vi "Protocol.Process Incoming Messages by PDU F.vi"(6 "State":T1=enum."ACL", 8 "error in":errorcluster, 10 "CAN frame":T2 {"payload" format="%x"; "timestamp" format="%<%.7X\n%x>T"; "type" items=["CAN Data"=0, "CAN Remote"=1, "CAN Bus Error"=2, "CAN 2.0 Data"=8, "CAN FD Data"=16, "CAN FD+BRS Data"=24, "J1939 Data"=192, "Delay"=224, "Log Trigger"=225, "Start Trigger"=226]; "identifier" format="%x"}, 11 "J1939 Cluster":T4) -> (0 "error out":errorcluster)   [LabVIEW 2023, in "J1939 Addon Engine.lvlib"]
uses:
  J1939 Addon Engine.lvlib
  Types/Protocol.Refs.ctl
  Support Libraries/J1939 Utilities/Types/CAN Outgoing Message Cluster.ctl
  Types/Protocol.RQST Lookup Table Reference.ctl
  Types/Protocol.Address Table Reference.ctl
  <vilib>/xnet/xnet.llb/XNET Frame CAN.ctl
  <vilib>/xnet/xnet.llb/XNET Frame Type CAN.ctl
  Support Libraries/J1939 Utilities/Types/Message Types.ctl
  Types/Protocol.RQST Lookup Table Action.ctl
  Types/Engine.Node DTC Settings.ctl
  Addon Shared/Types/Monitor Settings.ctl
  Types/Engine.DTC Settings.ctl
  Addon Shared/Types/Compiled Simulated Settings.ctl
  <vilib>/NI VeriStand/Custom Device API/Block Data Reference.ctl
  <vilib>/NI VeriStand/Custom Device API/Data Reference.ctl
  Types/Engine.DTC FIFOs.ctl
  Support Libraries/J1939 Utilities/Types/PGN Fields Cluster.ctl
  Types/Protocol.Address Lookup Table Action.ctl
  Addon Shared/Types/Address Lookup Table Data.ctl
  Support Libraries/J1939 Utilities/SubVIs/Convert CAN Arb ID to J1939 ID.vi
  Support Libraries/J1939 Utilities/SubVIs/Convert J1939 ID to CAN Arb ID.vi
  Support Libraries/J1939 Utilities/SubVIs/Convert CAN Data (U32) to U8.vi
  Support Libraries/J1939 Utilities/SubVIs/Acknowledgement.vi
  Protocol.Convert Data to DTC Frame.vi
  Protocol.RQST Lookup Table.vi
  <vilib>/xnet/xnet.llb/XNET Create Session.vi
  <vilib>/xnet/xnet.llb/XNET Create Session (Conversion).vi
  <vilib>/xnet/xnet.llb/XNET Convert.vi
  <vilib>/xnet/xnet.llb/XNET Convert (Signal to Frame CAN).vi
  <vilib>/xnet/xnet.llb/XNET Clear.vi
  Protocol.Address Lookup Table.vi
  Support Libraries/J1939 Utilities/J1939 Utilities.lvlib
  <vilib>/NI VeriStand/Custom Device API/Custom Device API.lvlib
  Addon Shared/J1939 Addon Shared.lvlib
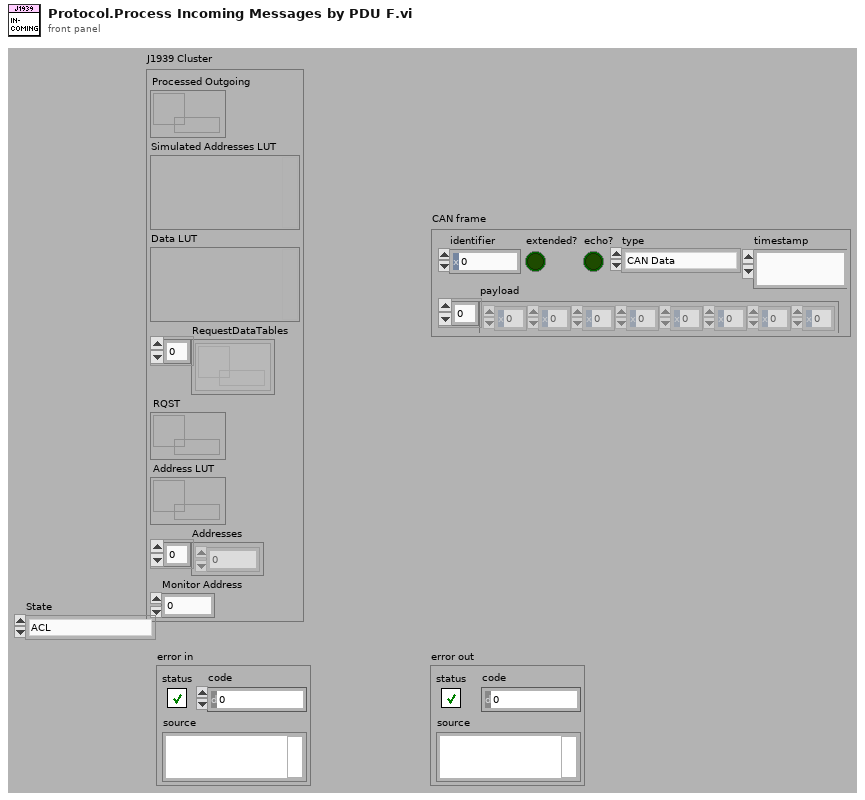
[diagram p1: front panel]
types:
  T1 = typedef "J1939 Utilities.lvlib/Message Types.ctl" = enum8{"PDU 1", "RQST2", "XFER", "ACKM", "RQST", "TP.DT - RTS/CTS", "TP.DT - BAM", "TP.CM - RTS", "TP.CM - CTS", "TP.CM - EndofMsgACK", "TP.CM - BAM", "TP.CM - Abort", "TP.CM - Error", "ACL", "Proprietary A", "PDU 2", "Proprietary B", "Error"}
  T2 = typedef "XNET Frame CAN.ctl" = cluster{"timestamp":timestamp, "payload":u8[], "identifier":u32, "type":T3, "extended?":bool, "echo?":bool}
  T3 = typedef "XNET Frame Type CAN.ctl" = u8
  T4 = typedef "J1939 Addon Engine.lvlib/Protocol.Refs.ctl" = cluster{"Processed Outgoing":refnum<queue>, "Simulated Addresses LUT":variant, "Data LUT":variant, "RequestDataTables":refnum<k33>[], "RQST":T5, "Address LUT":T6, "Addresses":u8[], "Monitor Address":u8}
  T5 = typedef "J1939 Addon Engine.lvlib/Protocol.RQST Lookup Table Reference.ctl" = refnum<data-value>
  T6 = typedef "J1939 Addon Engine.lvlib/Protocol.Address Table Reference.ctl" = refnum<data-value>
  T7 = typedef "J1939 Addon Engine.lvlib/Protocol.RQST Lookup Table Action.ctl" = enum16{"Initialize", "Add", "Get", "Remove", "Get Active Requests"}
  T8 = typedef "J1939 Addon Engine.lvlib/Engine.Node DTC Settings.ctl" = cluster{"Network":T9, "Sim DTC Refs":T10}
  T9 = typedef "J1939 Addon Shared.lvlib/Monitor Settings.ctl" = cluster{"Address":u8, "Name":u64, "Include DA":bool, "Force SA":bool}
  T10 = typedef "J1939 Addon Engine.lvlib/Engine.DTC Settings.ctl" = cluster{"Data":T11, "FIFOs":T14}
  T11 = typedef "J1939 Addon Shared.lvlib/Compiled Simulated Settings.ctl" = cluster{"DM1.Ref":T12[], "DM1.Value":dbl[], "DM1.Enable.Ref":T12[], "DM1.Enable.Value":dbl[], "DM2.Ref":T12[], "DM2.Value":dbl[], "DM2.Enable.Ref":T12[], "DM2.Enable.Value":dbl[]}
  T12 = typedef "Custom Device API.lvlib/Block Data Reference.ctl" = cluster{"Data Reference":T13, "Offset":u64, "Length":u64}
  T13 = typedef "Custom Device API.lvlib/Data Reference.ctl" = i32
  T14 = typedef "J1939 Addon Engine.lvlib/Engine.DTC FIFOs.ctl" = cluster{"DM1.Data":refnum<k33>, "DM1.Enable":refnum<k33>, "DM2.Data":refnum<k33>, "DM2.Enable":refnum<k33>, "DM1.Reset":refnum<k33>, "DM2.Reset":refnum<k33>}
  T15 = typedef "J1939 Utilities.lvlib/PGN Fields Cluster.ctl" = cluster{"Reserved Bit":u8, "Data page":u8, "PDU Format":u8, "PDU Specific":u8}
  T16 = typedef "J1939 Utilities.lvlib/CAN Outgoing Message Cluster.ctl" = cluster{"Identifier":u32, "Data":u8[]}
  T17 = typedef "J1939 Addon Engine.lvlib/Protocol.Address Lookup Table Action.ctl" = enum16{"Initialize", "Add", "Get", "Remove", "Get All"}
  T18 = typedef "J1939 Addon Shared.lvlib/Address Lookup Table Data.ctl" = cluster{"Name":u8[], "Address":u8}
  T19 = typedef "J1939 Addon Engine.lvlib/Protocol.RQST Lookup Table Cluster.ctl" = cluster{"Response Q":refnum<queue>, "Request PGN":u32}
  T20 = typedef "J1939 Utilities.lvlib/Convert CAN Data (U8) Cluster.ctl" = cluster{"Byte 1":u8, "Byte 2":u8, "Byte 3":u8, "Byte 4":u8, "Byte 5":u8, "Byte 6":u8, "Byte 7":u8, "Byte 8":u8}
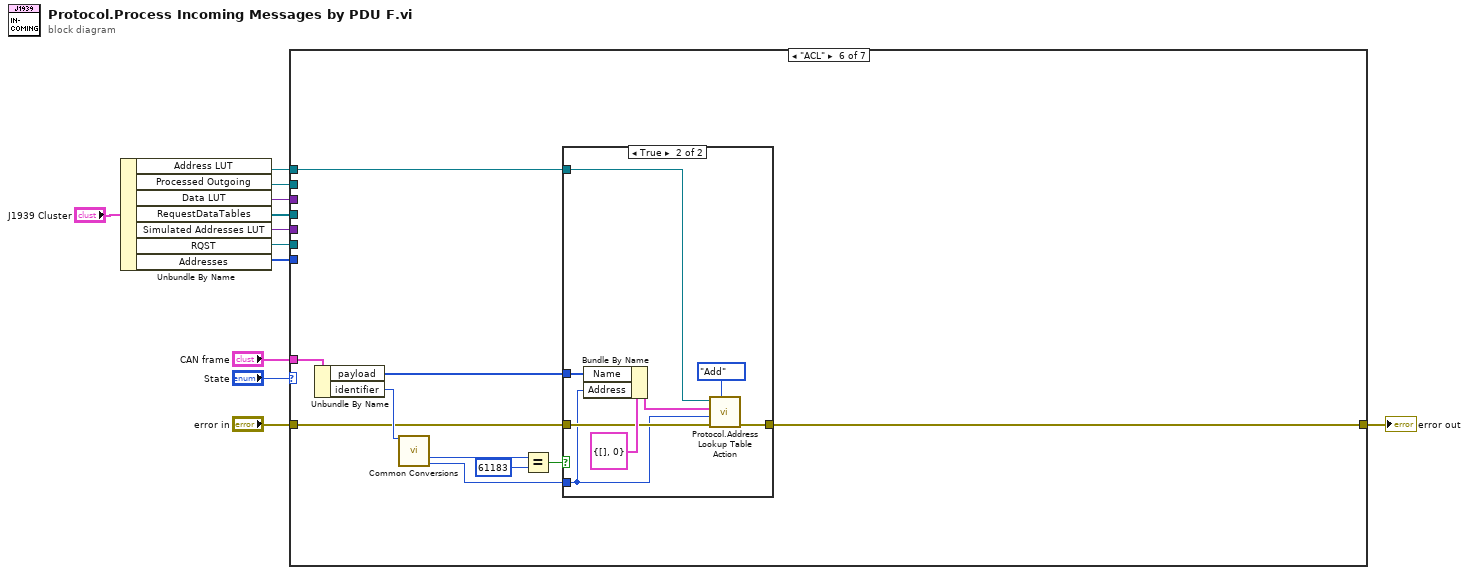
[diagram p0: block diagram]
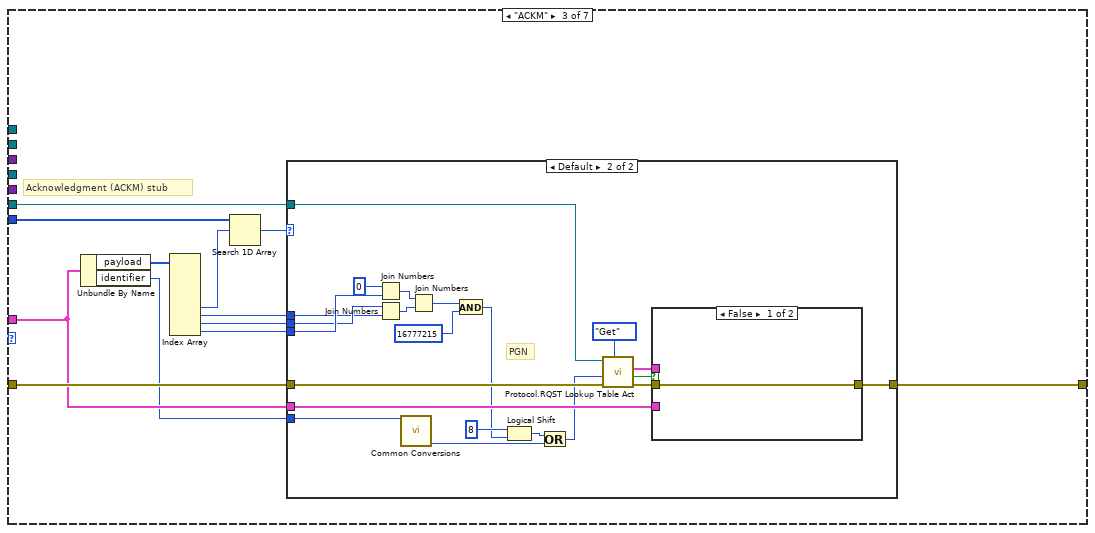
[diagram p4: hidden frame]
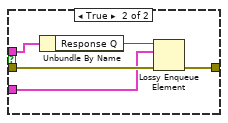
[diagram p6: hidden frame]
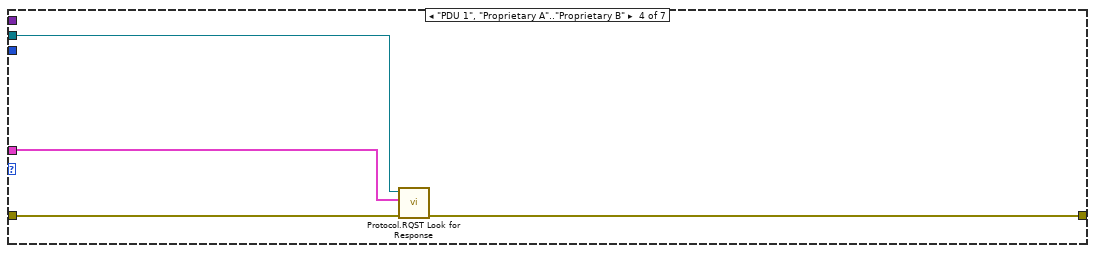
[diagram p7: hidden frame]
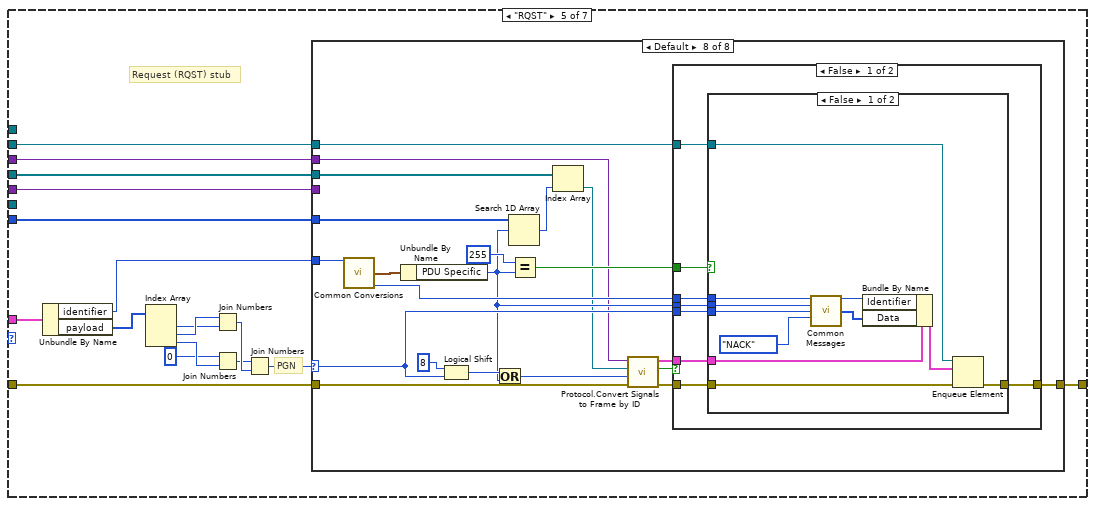
[diagram p8: hidden frame]
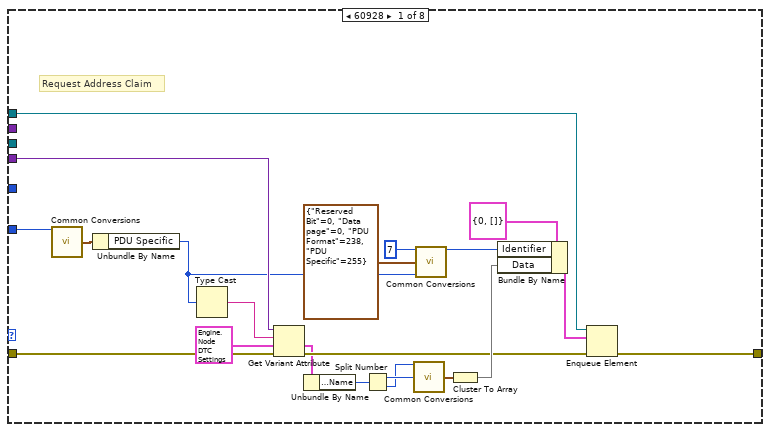
[diagram p9: hidden frame]
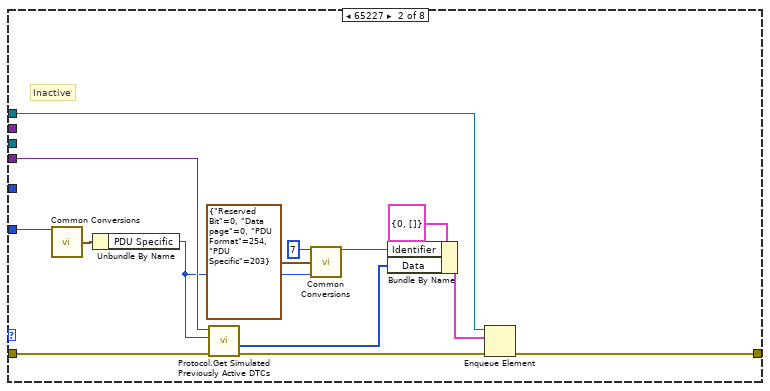
[diagram p10: hidden frame]
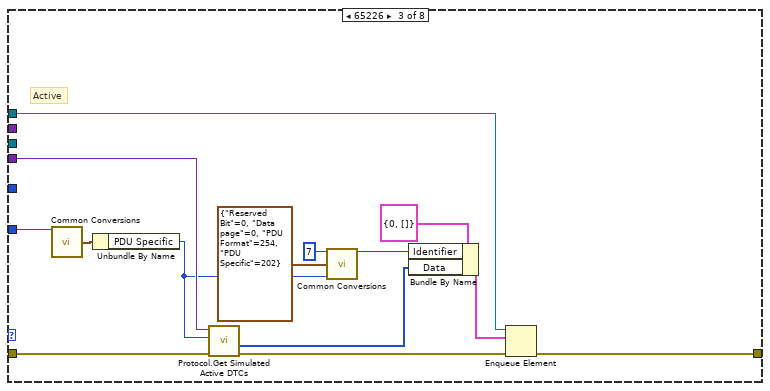
[diagram p11: hidden frame]
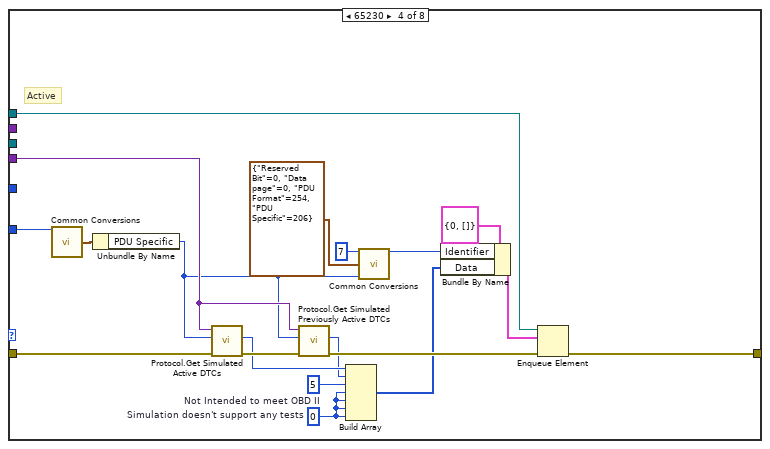
[diagram p12: hidden frame]
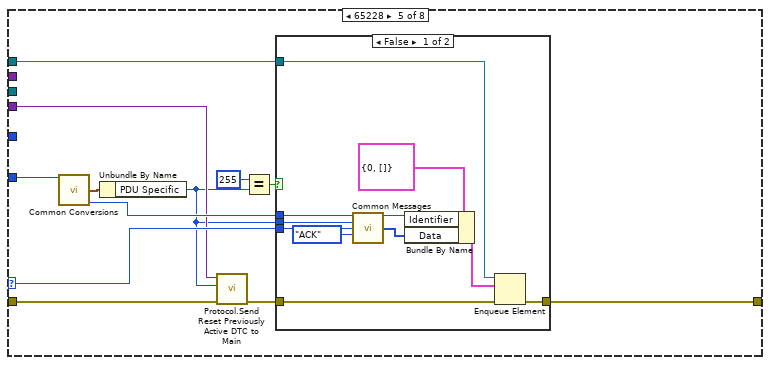
[diagram p13: hidden frame]
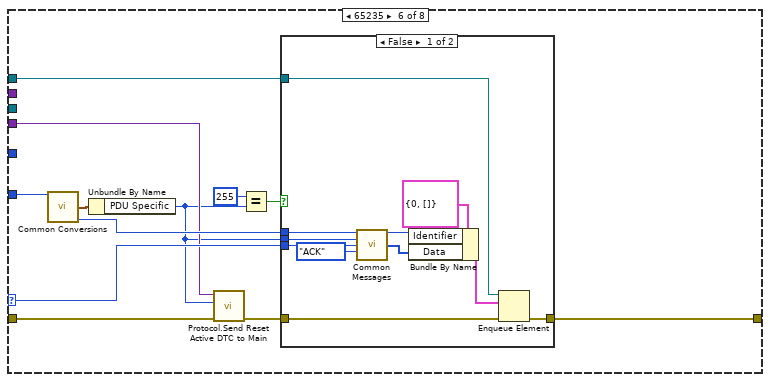
[diagram p15: hidden frame]
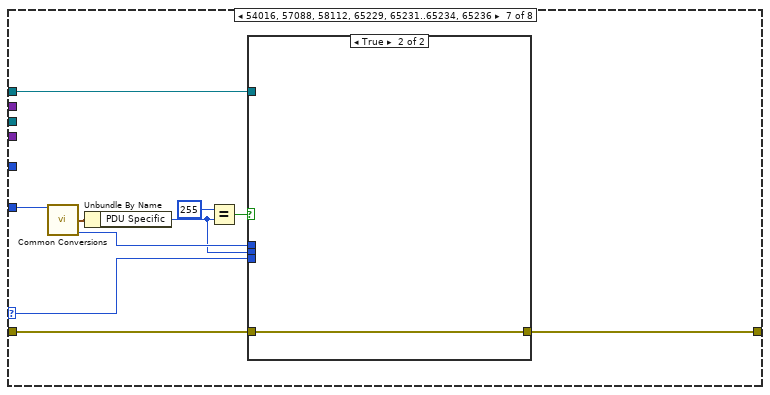
[diagram p17: hidden frame]
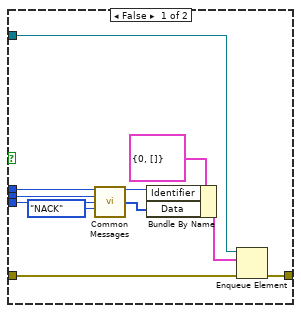
[diagram p18: hidden frame]
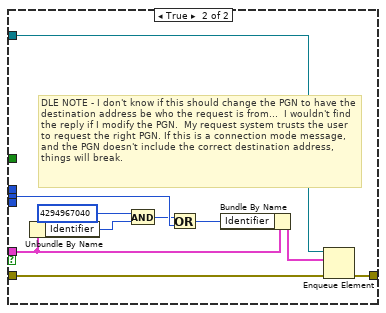
[diagram p20: hidden frame]
diagram:
  n1 = Unbundle By Name("J1939 Cluster") -> ("Address LUT"=w1:T6, "Processed Outgoing"=w6:refnum<queue>, "Data LUT"=w9:variant, "RequestDataTables"=w8:refnum<k33>[], "Simulated Addresses LUT"=w7:variant, "RQST"=w10:T5, "Addresses"=w5:u8[])
  n2 = case shown="\"ACL\"" "State" {
    tunnel: "error in" -> [w13 w14 w21 w59 w67 w269 w285]
    tunnel: [w13 w14 w22 w57 w68 w268 w285] -> w12
    tunnel: "CAN frame" -> [_ _ w20 w58 w76 w270 _]
    tunnel: w6 -> [_ _ _ _ w66 _ _]
    tunnel: w10 -> [_ _ w18 w56 _ _ _]
    tunnel: w5 -> [_ _ w17 _ w61 _ _]
    tunnel: w7 -> [_ _ _ _ w63 _ _]
    tunnel: w8 -> [_ _ _ _ w62 _ _]
    tunnel: w9 -> [_ _ _ _ w60 _ _]
    tunnel: w1 -> [_ _ _ _ _ w266 _]
    frame "RQST2" {
      # "Request2 (RQST2) Stub"
    }
    frame "XFER" {
      # "Transfer (XFER) Stub"
    }
    frame "ACKM" {
      # "Acknowledgment (ACKM) stub"
      n3 = Unbundle By Name(w20) -> ("payload"=w26:u8[], "identifier"=w19:u32)
      n4 = Index Array(array=w26) -> (element #5=w16:u8, element #6=w23:u8, element #7=w24:u8, element #8=w25:u8)  [unwired: 8 in, 4 out]
      n5 = Search 1D Array(1D array=w17, element=w16) -> (index of element=w15:i32)  [unwired: 1 in]
      n6 = case shown="Default" w15 {
        tunnel: w25 -> [_ w49]
        tunnel: w24 -> [_ w48]
        tunnel: w23 -> [_ w47]
        tunnel: [w27 w39] -> w22
        tunnel: w21 -> [w27 w38]
        tunnel: w20 -> [_ w37]
        tunnel: w19 -> [_ w34]
        tunnel: w18 -> [_ w29]
        frame -1 {
        }
        frame Default {
          # "PGN"
          n7 = Join Numbers(hi=u8 0, lo=w49) -> ((hi.lo)=w46:u16)
          n8 = Join Numbers(hi=w48, lo=w47) -> ((hi.lo)=w45:u16)
          n9 = call-poly "Common Conversions.vi"("Arb ID"=w34) -> ("Source Address"=w33:u8)  [unwired: 11 in, 3 out]
          n10 = Join Numbers(hi=w46, lo=w45) -> ((hi.lo)=w44:u32)
          n11 = And(x=w44, y=u32 16777215 ("x")) -> (x .and. y?=w32:u32)
          n12 = Logical Shift(y=i8 8, x=w32) -> (x << y=w36:u32)
          n13 = Or(x=w36, y=w33) -> (x .or. y?=w31:u32)
          n14 = call "Protocol.RQST Lookup Table Act.vi"("Action"=Protocol.RQST_Lookup_Table_Action."Get", "error in (no error)"=w38, "ID"=w31, "Rqst LUT"=w29) -> ("error out"=w30:errorcluster, "Found?"=w41:bool, "Data"=w40:T19)  [unwired: 3 in, 2 out]
          n15 = case shown="False" w41 {
            tunnel: w40 -> [_ w54]
            tunnel: w30 -> [w50 w55]
            tunnel: w37 -> [_ w52]
            tunnel: [w50 w51] -> w39
            frame False {
            }
            frame True {
              n16 = Unbundle By Name(w54) -> ("Response Q"=w53:refnum<queue>)
              n17 = Lossy Enqueue Element(queue=w53, element=w52, error in (no error)=w55) -> (error out=w51:errorcluster)  [unwired: 3 out]
            }
          }
        }
      }
    }
    frame "PDU 1", "Proprietary A".."Proprietary B" {
      n18 = call "Protocol.RQST Look for Response.vi"("error in (no error)"=w59, "CAN frame"=w58, "ref in"=w56) -> ("error out"=w57:errorcluster)  [unwired: 8 in]
    }
    frame "RQST" {
      # "PGN"
      # "Request (RQST) stub"
      n19 = Unbundle By Name(w76) -> ("identifier"=w65:u32, "payload"=w75:u8[])
      n20 = Index Array(array=w75) -> (element #1=w64:u8, element #2=w74:u8, element #3=w73:u8)  [unwired: 3 in]
      n21 = Join Numbers(hi=w74, lo=w64) -> ((hi.lo)=w71:u16)
      n22 = Join Numbers(hi=u8 0, lo=w73) -> ((hi.lo)=w70:u16)
      n23 = Join Numbers(hi=w70, lo=w71) -> ((hi.lo)=w69:u32)
      n24 = case shown="Default" w69 {
        selector: w69 -> [_ _ _ _ w150 w175 w197 w227]
        tunnel: [w93 w104 w119 w138 w151 w173 w195 w228] -> w68
        tunnel: w67 -> [w81 w100 w113 w135 w148 w170 w193 w235]
        tunnel: w66 -> [w91 w103 w118 w137 w152 w176 w198 w229]
        tunnel: w65 -> [w85 w110 w124 w143 w155 w174 w196 w230]
        tunnel: w63 -> [w83 w102 w115 w132 w146 w172 _ _]
        tunnel: w62 -> [_ _ _ _ _ _ _ w218]
        tunnel: w61 -> [_ _ _ _ _ _ _ w220]
        tunnel: w60 -> [_ _ _ _ _ _ _ w215]
        frame 60928 {
          # "Request Address Claim"
          n25 = call-poly "Common Conversions.vi"("Arb ID"=w85) -> ("PGN Fields"=w86:T15)  [unwired: 11 in, 3 out]
          n26 = Unbundle By Name(w86) -> ("PDU Specific"=w82:u8)
          n27 = Type Cast(x=w82) -> (*(type *) &x=w84:string)  [unwired: 1 in]
          n28 = Get Variant Attribute(Variant=w83, name=w84, default value (empty Variant)=T8 {"Network"={"Address"=0, "Name"=0, "Include DA"=FALSE, "Force SA"=FALSE}, "Sim DTC Refs"={"Data"={"DM1.Ref"=[], "DM1.Value"=[], "DM1.Enable.Ref"=[], "DM1.Enable.Value"=[], "DM2.Ref"=[], "DM2.Value"=[], "DM2.Enable.Ref"=[], "DM2.Enable.Value"=[]}, "FIFOs"={"DM1.Data"=refnum, "DM1.Enable"=refnum, "DM2.Data"=refnum, "DM2.Enable"=refnum, "DM1.Reset"=refnum, "DM2.Reset"=refnum}}} ("cluster"), error in=w81) -> (value=w79:T8, error out=w80:errorcluster)  [unwired: 2 out]
          n29 = Unbundle By Name(w79) -> ("Network.Name"=w78:u64)
          n30 = Split Number(x=w78) -> (hi(x)=w89:u32, lo(x)=w88:u32)
          n31 = call-poly "Common Conversions.vi"("Data 0-3"=w88, "Data 4-7"=w89) -> ("Byte Cluster"=w90:T20)  [unwired: 13 in]
          n32 = call-poly "Common Conversions.vi"("Priority"=u8 7, "PGN Fields"=T15 {"Reserved Bit"=0, "Data page"=0, "PDU Format"=238, "PDU Specific"=255}, "Source Address"=w82) -> ("ID"=w95:u32)  [unwired: 2 in, 10 out]
          n33 = Cluster To Array(cluster=w90) -> (array=w87:u8[])
          n34 = Bundle By Name(cluster=T16 {"Identifier"=0, "Data"=[]} ("Data to Send"), "Identifier"=w95, "Data"=w87) -> (w92:T16)
          n35 = Enqueue Element(queue=w91, element=w92, error in (no error)=w80) -> (error out=w93:errorcluster)  [unwired: 1 in, 2 out]
        }
        frame 65227 {
          # "Inactive"
          n36 = call-poly "Common Conversions.vi"("Arb ID"=w110) -> ("PGN Fields"=w111:T15)  [unwired: 11 in, 3 out]
          n37 = Unbundle By Name(w111) -> ("PDU Specific"=w101:u8)
          n38 = call "Protocol.Get Simulated Previously Active DTCs.vi"("error in (no error)"=w100, "Address"=w101, "Simulated Addresses LUT"=w102) -> ("error out"=w99:errorcluster, "DTC Frame"=w98:u8[])  [unwired: 5 in, 2 out]
          n39 = call-poly "Common Conversions.vi"("Priority"=u8 7, "PGN Fields"=T15 {"Reserved Bit"=0, "Data page"=0, "PDU Format"=254, "PDU Specific"=203}, "Source Address"=w101) -> ("ID"=w107:u32)  [unwired: 2 in, 10 out]
          n40 = Bundle By Name(cluster=T16 {"Identifier"=0, "Data"=[]} ("Data to Send"), "Identifier"=w107, "Data"=w98) -> (w109:T16)
          n41 = Enqueue Element(queue=w103, element=w109, error in (no error)=w99) -> (error out=w104:errorcluster)  [unwired: 1 in, 2 out]
        }
        frame 65226 {
          # "Active"
          n42 = call-poly "Common Conversions.vi"("Arb ID"=w124) -> ("PGN Fields"=w125:T15)  [unwired: 11 in, 3 out]
          n43 = Unbundle By Name(w125) -> ("PDU Specific"=w114:u8)
          n44 = call "Protocol.Get Simulated Active DTCs.vi"("error in (no error)"=w113, "Address"=w114, "Simulated Addresses LUT"=w115) -> ("error out"=w116:errorcluster, "DTC Frame"=w112:u8[])  [unwired: 5 in, 2 out]
          n45 = call-poly "Common Conversions.vi"("Priority"=u8 7, "PGN Fields"=T15 {"Reserved Bit"=0, "Data page"=0, "PDU Format"=254, "PDU Specific"=202}, "Source Address"=w114) -> ("ID"=w121:u32)  [unwired: 2 in, 10 out]
          n46 = Bundle By Name(cluster=T16 {"Identifier"=0, "Data"=[]} ("Data to Send"), "Identifier"=w121, "Data"=w112) -> (w123:T16)
          n47 = Enqueue Element(queue=w118, element=w123, error in (no error)=w116) -> (error out=w119:errorcluster)  [unwired: 1 in, 2 out]
        }
        frame 65230 {
          w128 = u8 0  # Simulation doesn't support any tests
          w129 = u8 5  # Not Intended to meet OBD II
          # "Active"
          n48 = call-poly "Common Conversions.vi"("Arb ID"=w143) -> ("PGN Fields"=w144:T15)  [unwired: 11 in, 3 out]
          n49 = Unbundle By Name(w144) -> ("PDU Specific"=w126:u8)
          n50 = call "Protocol.Get Simulated Active DTCs.vi"("error in (no error)"=w135, "Address"=w126, "Simulated Addresses LUT"=w132) -> ("error out"=w134:errorcluster, "# of Enabled"=w131:u8)  [unwired: 5 in, 2 out]
          n51 = call "Protocol.Get Simulated Previously Active DTCs.vi"("error in (no error)"=w134, "Address"=w126, "Simulated Addresses LUT"=w132) -> ("error out"=w133:errorcluster, "# of Enabled"=w130:u8)  [unwired: 5 in, 2 out]
          n52 = Build Array(w131, w130, w129, w128, w128, w128, w128) -> (w127:u8[])
          n53 = call-poly "Common Conversions.vi"("Priority"=u8 7, "PGN Fields"=T15 {"Reserved Bit"=0, "Data page"=0, "PDU Format"=254, "PDU Specific"=206}, "Source Address"=w126) -> ("ID"=w140:u32)  [unwired: 2 in, 10 out]
          n54 = Bundle By Name(cluster=T16 {"Identifier"=0, "Data"=[]} ("Data to Send"), "Identifier"=w140, "Data"=w127) -> (w142:T16)
          n55 = Enqueue Element(queue=w137, element=w142, error in (no error)=w133) -> (error out=w138:errorcluster)  [unwired: 1 in, 2 out]
        }
        frame 65228 {
          n56 = call-poly "Common Conversions.vi"("Arb ID"=w155) -> ("PGN Fields"=w156:T15, "Source Address"=w149:u8)  [unwired: 11 in, 2 out]
          n57 = Unbundle By Name(w156) -> ("PDU Specific"=w145:u8)
          n58 = call "Protocol.Send Reset Previously Active DTC to Main.vi"("error in (no error)"=w148, "Address"=w145, "Simulated Addresses LUT"=w146) -> ("error out"=w147:errorcluster)  [unwired: 7 in, 1 out]
          n59 = Equal?(x=u8 255 ("y"), y=w145) -> (x = y?=w153:bool)
          n60 = case shown="False" w153 {
            tunnel: w147 -> [w167 w168]
            tunnel: [w166 w168] -> w151
            tunnel: w152 -> [w165 _]
            tunnel: w149 -> [w164 _]
            tunnel: w145 -> [w163 _]
            tunnel: w150 -> [w162 _]
            frame False {
              n61 = call-poly "Common Messages.vi"("Destination Address"=w164, "Source Address"=w163, "PGN"=w162, "Control Byte"=enum8{"ACK", "NACK", "Access Denied"}."ACK") -> ("Arb ID"=w160:u32, "Data"=w159:u8[])  [unwired: 10 in]
              n62 = Bundle By Name(cluster=T16 {"Identifier"=0, "Data"=[]} ("Frame"), "Identifier"=w160, "Data"=w159) -> (w158:T16)
              n63 = Enqueue Element(queue=w165, element=w158, error in (no error)=w167) -> (error out=w166:errorcluster)  [unwired: 3 out]
            }
            frame True {
            }
          }
        }
        frame 65235 {
          n64 = call-poly "Common Conversions.vi"("Arb ID"=w174) -> ("PGN Fields"=w180:T15, "Source Address"=w177:u8)  [unwired: 11 in, 2 out]
          n65 = Unbundle By Name(w180) -> ("PDU Specific"=w171:u8)
          n66 = call "Protocol.Send Reset Active DTC to Main.vi"("error in (no error)"=w170, "Address"=w171, "Simulated Addresses LUT"=w172) -> ("error out"=w169:errorcluster)  [unwired: 7 in, 1 out]
          n67 = Equal?(x=u8 255 ("y"), y=w171) -> (x = y?=w178:bool)
          n68 = case shown="False" w178 {
            tunnel: w169 -> [w191 w192]
            tunnel: [w190 w192] -> w173
            tunnel: w176 -> [w189 _]
            tunnel: w177 -> [w188 _]
            tunnel: w171 -> [w187 _]
            tunnel: w175 -> [w186 _]
            frame False {
              n69 = call-poly "Common Messages.vi"("Destination Address"=w188, "Source Address"=w187, "PGN"=w186, "Control Byte"=enum8{"ACK", "NACK", "Access Denied"}."ACK") -> ("Arb ID"=w184:u32, "Data"=w183:u8[])  [unwired: 10 in]
              n70 = Bundle By Name(cluster=T16 {"Identifier"=0, "Data"=[]} ("Frame"), "Identifier"=w184, "Data"=w183) -> (w182:T16)
              n71 = Enqueue Element(queue=w189, element=w182, error in (no error)=w191) -> (error out=w190:errorcluster)  [unwired: 3 out]
            }
            frame True {
            }
          }
        }
        frame 54016, 57088, 58112, 65229, 65231..65234, 65236 {
          n72 = call-poly "Common Conversions.vi"("Arb ID"=w196) -> ("PGN Fields"=w202:T15, "Source Address"=w199:u8)  [unwired: 11 in, 2 out]
          n73 = Unbundle By Name(w202) -> ("PDU Specific"=w194:u8)
          n74 = Equal?(x=u8 255 ("y"), y=w194) -> (x = y?=w200:bool)
          n75 = case shown="True" w200 {
            tunnel: w193 -> [w213 w214]
            tunnel: [w212 w214] -> w195
            tunnel: w198 -> [w211 _]
            tunnel: w199 -> [w210 _]
            tunnel: w194 -> [w209 _]
            tunnel: w197 -> [w208 _]
            frame False {
              n76 = call-poly "Common Messages.vi"("Destination Address"=w210, "Source Address"=w209, "PGN"=w208, "Control Byte"=enum8{"ACK", "NACK", "Access Denied"}."NACK") -> ("Arb ID"=w206:u32, "Data"=w205:u8[])  [unwired: 10 in]
              n77 = Bundle By Name(cluster=T16 {"Identifier"=0, "Data"=[]} ("Frame"), "Identifier"=w206, "Data"=w205) -> (w204:T16)
              n78 = Enqueue Element(queue=w211, element=w204, error in (no error)=w213) -> (error out=w212:errorcluster)  [unwired: 3 out]
            }
            frame True {
            }
          }
        }
        frame Default {
          n79 = call-poly "Common Conversions.vi"("Arb ID"=w230) -> ("PGN Fields"=w226:T15, "Source Address"=w223:u8)  [unwired: 11 in, 2 out]
          n80 = Unbundle By Name(w226) -> ("PDU Specific"=w219:u8)
          n81 = Logical Shift(y=i8 8, x=w227) -> (x << y=w222:u32)
          n82 = Or(x=w222, y=w219) -> (x .or. y?=w221:u32)
          n83 = Search 1D Array(1D array=w220, element=w219) -> (index of element=w217:i32)  [unwired: 1 in]
          n84 = Equal?(x=u8 255 ("y"), y=w219) -> (x = y?=w224:bool)
          n85 = Index Array(array=w218, index=w217) -> (element=w216:refnum<k33>)
          n86 = call "Protocol.Convert Signals to Frame by ID.vi"("error in (no error)"=w235, "ID"=w221, "RequestDataTable"=w216, "Data LUT"=w215) -> ("error out"=w231:errorcluster, "Found?"=w232:bool, "Frame"=w233:T16)  [unwired: 5 in]
          n87 = case shown="False" w232 {
            tunnel: w233 -> [w237 w265]
            tunnel: w219 -> [w239 w263]
            tunnel: [w242 w258] -> w228
            tunnel: w231 -> [w243 w259]
            tunnel: w223 -> [w240 _]
            tunnel: w229 -> [w241 w260]
            tunnel: w227 -> [w238 _]
            tunnel: w224 -> [w236 _]
            frame False {
              n88 = case shown="False" w236 {
                tunnel: w243 -> [w254 w255]
                tunnel: [w253 w255] -> w242
                tunnel: w241 -> [w252 _]
                tunnel: w240 -> [w251 _]
                tunnel: w239 -> [w250 _]
                tunnel: w238 -> [w249 _]
                tunnel: w237 -> [w247 _]
                frame False {
                  n89 = call-poly "Common Messages.vi"("Destination Address"=w251, "Source Address"=w250, "PGN"=w249, "Control Byte"=enum8{"ACK", "NACK", "Access Denied"}."NACK") -> ("Arb ID"=w246:u32, "Data"=w245:u8[])  [unwired: 10 in]
                  n90 = Bundle By Name(cluster=w247, "Identifier"=w246, "Data"=w245) -> (w244:T16)
                  n91 = Enqueue Element(queue=w252, element=w244, error in (no error)=w254) -> (error out=w253:errorcluster)  [unwired: 3 out]
                }
                frame True {
                }
              }
            }
            frame True {
              # "DLE NOTE - I don't know if this should change the PGN to have the destination address be who the request is from...  I wouldn't find the reply if I modify the PGN.  My request system trusts the user to request the right PGN. If this is a connection mode message, and the PGN doesn't include the correct destination address, things will break."
              n92 = Unbundle By Name(w265) -> ("Identifier"=w264:u32)
              n93 = And(x=u32 4294967040 ("y"), y=w264) -> (x .and. y?=w256:u32)
              n94 = Or(x=w256, y=w263) -> (x .or. y?=w262:u32)
              n95 = Bundle By Name(cluster=w265, "Identifier"=w262) -> (w261:T16)
              n96 = Enqueue Element(queue=w260, element=w261, error in (no error)=w259) -> (error out=w258:errorcluster)  [unwired: 3 out]
            }
          }
        }
      }
    }
    frame "ACL" {
      n97 = Unbundle By Name(w270) -> ("payload"=w271:u8[], "identifier"=w275:u32)
      n98 = call-poly "Common Conversions.vi"("Arb ID"=w275) -> ("PGN"=w274:u32, "Source Address"=w272:u8)  [unwired: 11 in, 2 out]
      n99 = Equal?(x=w274, y=u32 61183) -> (x = y?=w267:bool)
      n100 = case shown="True" w267 {
        tunnel: w272 -> [_ w278]
        tunnel: w271 -> [_ w284]
        tunnel: w269 -> [w276 w281]
        tunnel: [w276 w280] -> w268
        tunnel: w266 -> [_ w279]
        frame False {
        }
        frame True {
          n101 = Bundle By Name(cluster=T18 {"Name"=[], "Address"=0} ("Data"), "Name"=w284, "Address"=w278) -> (w282:T18)
          n102 = call "Protocol.Address Lookup Table Action.vi"("Action"=Protocol.Address_Lookup_Table_Action."Add", "error in (no error)"=w281, "Address"=w278, "Data"=w282, "ref in"=w279) -> ("error out"=w280:errorcluster)  [unwired: 3 in, 3 out]
        }
      }
    }
    frame "Error", Default {
    }
  }
  "error out" <- w12
